vi "Init Arm Zero.vi"(1 "error in":errorcluster) -> (0 "error out":errorcluster)   [LabVIEW 2020]
uses:
  Global Arm Variables.vi
panel:
  out "pottValueForArmAtZeroDegrees":sgl
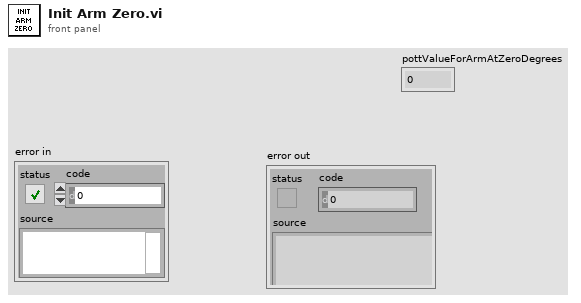
[diagram p1: front panel]
types:
  T1 = typedef "WPI_PotentiometerDevRef.ctl" = cluster{"DevStatus":errorcluster, "Analog Channel":T2, "Invert Output":bool}
  T2 = typedef "FPGA_AIChannel.ctl" = enum8{"AI 0", "AI 1", "AI 2", "AI 3", "AI MXP 0", "AI MXP 1", "AI MXP 2", "AI MXP 3", "Invalid"}
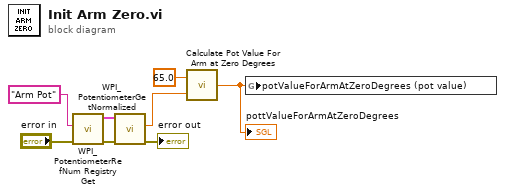
[diagram p0: block diagram]
diagram:
  n1 = call <vilib>:"WPI_PotentiometerRefNum Registry Get.vi"("error in (no error)"="error in", "refnum name"="Arm Pot") -> ("error out"=w3:errorcluster, "PotDevRef"=w8:T1)  [unwired: 8 in]
  n2 = call <vilib>:"WPI_PotentiometerGetNormalized.vi"("error in"=w3, "PotDevRef"=w8) -> ("error out"=→"error out":errorcluster, "Normalized Value"=w5:dbl)  [unwired: 7 in, 1 out]
  n3 = call "Calculate Pot Value For Arm at Zero Degrees.vi"("potValue"=w5, "arm Angle (degrees)"=65.0) -> ("pottValueForArmAtZeroDegrees"=w7:sgl)
  "pottValueForArmAtZeroDegrees" <- w7
  n4 = global write "Global Arm Variables.vi" "potValueForArmAtZeroDegrees (pot value)"(w7) -> ()
